vi "mav_main_mortar.vi"(8 "error in":errorcluster) -> (0 "error out":errorcluster)   [LabVIEW 2023]
uses:
  Global 1.vi
panel:
  out "logical OR":bool
  out "result":bool
  out "mortar_stage 2":T1
  in  "Connection Type":enum32{"TCP", "SERIAL", "UDP"}(tab)
  in  "tcp":cluster{"address":string, "port":u16}={"address"="192.168.2.101", "port"=2100}
  in  "serial":T2={"baudrate"=115200, "visa in"=""}
  in  "udp":cluster{"address":string, "port":u16}={"address"="127.0.0.1", "port"=5762}
  in  "stop":bool
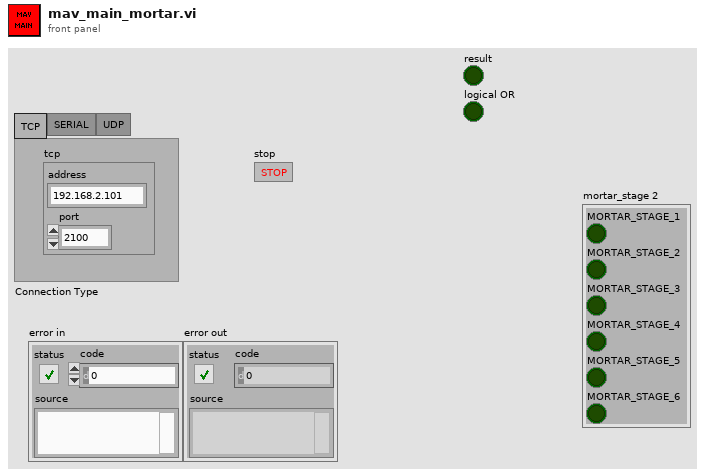
[diagram p1: front panel]
types:
  T1 = cluster{"MORTAR_STAGE_1":bool, "MORTAR_STAGE_2":bool, "MORTAR_STAGE_3":bool, "MORTAR_STAGE_4":bool, "MORTAR_STAGE_5":bool, "MORTAR_STAGE_6":bool}
  T2 = cluster{"baudrate":u32, "visa in":refnum<visa-resource-name>}
  T3 = cluster{"serial":cluster{"baudrate":u32, "visa in":refnum<visa-resource-name>}, "tcp":cluster{"address":string, "port":u16}, "udp":cluster{"address":string, "port":u16}}
  T4 = cluster{"visa out":refnum<visa-resource-name>, "tcp connection ID":refnum<k5>, "udp connection ID":refnum<k16>}
  T5 = cluster{"mortar_stage":cluster{"MORTAR_STAGE_1":bool, "MORTAR_STAGE_2":bool, "MORTAR_STAGE_3":bool, "MORTAR_STAGE_4":bool, "MORTAR_STAGE_5":bool, "MORTAR_STAGE_6":bool}, "target_system":u8, "target_component":u8, "self":cluster{"system_id":u8, "component_id":u8}}
  T6 = cluster{"len":u8, "incompat_flags":u8, "compat_flags":u8, "seq":u8, "sysid":u8, "compid":u8, "msgid":u32, "magic":u8, "payload":string, "checksum":u16, "signature":string}
  T7 = cluster{"time_usec":u32, "port":u8, "servo1_raw":u16, "servo2_raw":u16, "servo3_raw":u16, "servo4_raw":u16, "servo5_raw":u16, "servo6_raw":u16, "servo7_raw":u16, "servo8_raw":u16, "servo9_raw":u16, "servo10_raw":u16, "servo11_raw":u16, "servo12_raw":u16, "servo13_raw":u16, "servo14_raw":u16, "servo15_raw":u16, "servo16_raw":u16}
  T8 = cluster{"VISA out":refnum<visa-resource-name>, "tcp connection ID":refnum<k5>, "udp connection ID":refnum<k16>}
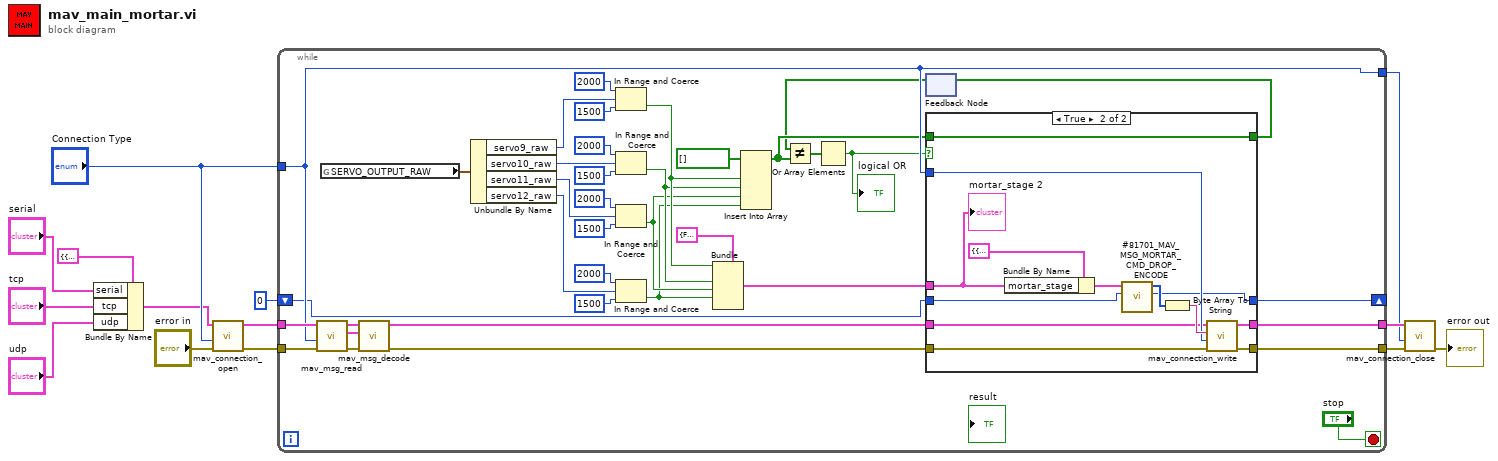
[diagram p0: block diagram]
diagram:
  n1 = Bundle By Name(cluster=T3 {"serial"={"baudrate"=115200, "visa in"=""}, "tcp"={"address"="127.0.0.1", "port"=5760}, "udp"={"address"="127.0.0.1", "port"=5760}} ("mav_connection_in"), "serial"="serial", "tcp"="tcp", "udp"="udp") -> (w2:T3)
  n2 = call "mav_connection_open.vi"("error in"="error in", "Connection Type"="Connection Type", "mav_connection_in"=w2) -> ("error out"=w9:errorcluster, "mav_connection_out"=w10:T4)  [unwired: 7 in]
  n3 = while {
    tunnel: "Connection Type" -> [w30]
    tunnel: [w26] -> w14
    tunnel: [w27] -> w13
    tunnel: [w30] -> w4
    tunnel: w9 -> [w47]
    tunnel: w10 -> [w48]
    shift-right: [w25] -> _
    shift-left: u8 0 ("packet_sequence_in") -> [w28]
    stop <- "stop" stop-if-true
    n4 = call "mav_msg_read.vi"("error in"=w47, "Connection Type"=w30, "mav_connection_in"=w48) -> ("error out"=w49:errorcluster, "mav_msg"=w50:T6, "mav_connection_out"=w51:T4)  [unwired: 6 in]
    n5 = global read "Global 1.vi" "SERVO_OUTPUT_RAW"() -> (w46:T7)
    n6 = call "mav_msg_decode.vi"("mav_connection_in"=w51, "mav_msg"=w50, "error in"=w49) -> ("mav_connection_out"=w29:T8, "error out"=w31:errorcluster)  [unwired: 6 in]
    n7 = Unbundle By Name(w46) -> ("servo9_raw"=w41:u16, "servo10_raw"=w42:u16, "servo11_raw"=w43:u16, "servo12_raw"=w44:u16)
    n8 = In Range and Coerce(upper limit=u16 2000, x=w41, lower limit=u16 1500) -> (In Range?=w24:bool)  [unwired: 1 out]
    n9 = In Range and Coerce(upper limit=u16 2000, x=w42, lower limit=u16 1500) -> (In Range?=w23:bool)  [unwired: 1 out]
    n10 = In Range and Coerce(upper limit=u16 2000, x=w43, lower limit=u16 1500) -> (In Range?=w22:bool)  [unwired: 1 out]
    n11 = In Range and Coerce(upper limit=u16 2000, x=w44, lower limit=u16 1500) -> (In Range?=w21:bool)  [unwired: 1 out]
    n12 = Bundle(cluster=T1 {"MORTAR_STAGE_1"=FALSE, "MORTAR_STAGE_2"=FALSE, "MORTAR_STAGE_3"=FALSE, "MORTAR_STAGE_4"=FALSE, "MORTAR_STAGE_5"=FALSE, "MORTAR_STAGE_6"=FALSE} ("mortar_stage 2"), "MORTAR_STAGE_1"=w24, "MORTAR_STAGE_3"=w23, "MORTAR_STAGE_4"=w22, "MORTAR_STAGE_5"=w21) -> (w32:T1)  [unwired: 2 in]
    n13 = Insert Into Array(array=bool[] [], new element #1=w24, new element #2=w23, new element #3=w22, new element #4=w21) -> (w19:bool[])  [unwired: 1 in]
    n14 = feedback #1() -> (w15:bool[])  [unwired: 1 in]
    n15 = Not Equal?(x=w15, y=w19) -> (x != y?=w18:bool[])
    n16 = Or Array Elements(Boolean array=w18) -> (logical OR=w17:bool)
    "logical OR" <- w17
    n17 = case shown="True" w17 {
      tunnel: w32 -> [_ w61]
      tunnel: w31 -> [w54 w66]
      tunnel: w30 -> [_ w65]
      tunnel: w29 -> [w55 w64]
      tunnel: w28 -> [w56 w63]
      tunnel: [w54 w60] -> w27
      tunnel: [w55 w59] -> w26
      tunnel: [w56 w58] -> w25
      tunnel: w19 -> [w53 w57]
      tunnel: [w53 w57] -> w16
      frame False {
      }
      frame True {
        n18 = Bundle By Name(cluster=T5 {"mortar_stage"={"MORTAR_STAGE_1"=TRUE, "MORTAR_STAGE_2"=TRUE, "MORTAR_STAGE_3"=TRUE, "MORTAR_STAGE_4"=TRUE, "MORTAR_STAGE_5"=TRUE, "MORTAR_STAGE_6"=TRUE}, "target_system"=1, "target_component"=50, "self"={"system_id"=1, "component_id"=50}} ("MORTAR_CMD_DROP"), "mortar_stage"=w61) -> (w67:T5)
        n19 = call "#81701_MAV_MSG_MORTAR_CMD_DROP_ENCODE.vi"("packet_sequence_in"=w63, "MORTAR_CMD_DROP"=w67) -> ("packet_sequence_out"=w58:u8, "mavlink_buffer_out"=w68:u8[])  [unwired: 8 in]
        n20 = Byte Array To String(unsigned byte array=w68) -> (string=w69:string)
        n21 = call "mav_connection_write.vi"("error in"=w66, "Connection Type"=w65, "data in"=w69, "mav_connection_in"=w64) -> ("error out"=w60:errorcluster, "mav_connection_out"=w59:T8)  [unwired: 6 in]
        "mortar_stage 2" <- w61
      }
    }
    n22 = feedback-in #1(w16) -> ()
  }
  n23 = call "mav_connection_close.vi"("error in"=w13, "Connection Type"=w4, "mav_connection_in"=w14) -> ("error out"=→"error out":errorcluster)  [unwired: 8 in]
